vi "execute_trajectory_segment_final_point_only.vi"(6 "end time override":dbl=0.5, 8 "error in":errorcluster, 10 "in PathPlannerWayPoints":T1[](array[typedef]) {"HolonomicRotation"."SIN" format="%13.4f"; "HolonomicRotation"."COS" format="%13.4f"; "HolonomicRotation"."VALUE" format="%13.4f"; "NextControl"."Y" format="%14.3f"; "NextControl"."X" format="%14.3f"; "PrevControl"."Y" format="%14.3f"; "PrevControl"."X" format="%14.3f"; "AnchorPoint"."Y" format="%14.3f"; "AnchorPoint"."X" format="%14.3f"}, 11 "inHOLONOMIC_DRV_CTRL":T4={"poseTolerance"={"TRANSLATION"={"X"=0.0, "Y"=0.0}, "ROTATION"={"VALUE"=0.0, "COS"=1.0, "SIN"=0.0}}, "poseError"={"TRANSLATION"={"X"=0.0, "Y"=0.0}, "ROTATION"={"VALUE"=0.0, "COS"=1.0, "SIN"=0.0}}, "Enabled"=TRUE, "PID_xCtrl"={"Kp"=0.0, "Ki"=0.0, "Kd"=0.0, "Period"=0.0, "Max_Integral"=1.0, "Min_Integral"=-1.0, "Max_Input"=0.0, "Min_Input"=0.0, "Continuous"=FALSE, "PositionError"=0.0, "VelocityError"=0.0, "PrevError"=0.0, "TotalError"=0.0, "PositionTolerance"=0.05, "VelocityTolerance"=9.99e+35, "SetPoint"=0.0, "Kf"=0.0, "Prev_Deriv"=0.0, "Prev_Deriv 2"=0.0, "DerivativeFilter"=FALSE, "Min_Output"=-9.99e+35, "Max_Output"=9.9e+35, "Prev_F_P"=0.0, "Prev_F_P_2"=0.0, "AntiWindupActive"=FALSE, "Measurement"=0.0}, "PID_yCtrl"={"Kp"=0.0, "Ki"=0.0, "Kd"=0.0, "Period"=0.0, "Max_Integral"=1.0, "Min_Integral"=-1.0, "Max_Input"=0.0, "Min_Input"=0.0, "Continuous"=FALSE, "PositionError"=0.0, "VelocityError"=0.0, "PrevError"=0.0, "TotalError"=0.0, "PositionTolerance"=0.05, "VelocityTolerance"=9.99e+35, "SetPoint"=0.0, "Kf"=0.0, "Prev_Deriv"=0.0, "Prev_Deriv 2"=0.0, "DerivativeFilter"=FALSE, "Min_Output"=-9.99e+35, "Max_Output"=9.9e+35, "Prev_F_P"=0.0, "Prev_F_P_2"=0.0, "AntiWindupActive"=FALSE, "Measurement"=0.0}, "PROF_PID_thetaCtrl"={"Controller"={"Kp"=0.0, "Ki"=0.0, "Kd"=0.0, "Period"=0.0, "Max_Integral"=1.0, "Min_Integral"=-1.0, "Max_Input"=0.0, "Min_Input"=0.0, "Continuous"=FALSE, "PositionError"=0.0, "VelocityError"=0.0, "PrevError"=0.0, "TotalError"=0.0, "PositionTolerance"=0.05, "VelocityTolerance"=9.99e+35, "SetPoint"=0.0, "Kf"=0.0, "Prev_Deriv"=0.0, "Prev_Deriv 2"=0.0, "DerivativeFilter"=FALSE, "Min_Output"=-9.99e+35, "Max_Output"=9.9e+35, "Prev_F_P"=0.0, "Prev_F_P_2"=0.0, "AntiWindupActive"=FALSE, "Measurement"=0.0}, "Goal"={"Position"=0.0, "Velocity"=0.0}, "Setpoint"={"Position"=0.0, "Velocity"=0.0}, "Constraint"={"MaxVelocity"=0.0, "MaxAcceleration"=0.0}}, "RotationError"={"VALUE"=0.0, "COS"=1.0, "SIN"=0.0}, "FirstRun"=TRUE} {"RotationError"."SIN" format="%13.4f"; "RotationError"."COS" format="%13.4f"; "RotationError"."VALUE" format="%13.4f"; "PROF_PID_thetaCtrl"."Constraint"."MaxAcceleration" format="%16_6e"; "PROF_PID_thetaCtrl"."Constraint"."MaxVelocity" format="%16_6e"; "PROF_PID_thetaCtrl"."Setpoint"."Velocity" format="%16_6e"; "PROF_PID_thetaCtrl"."Setpoint"."Position" format="%16_6e"; "PROF_PID_thetaCtrl"."Goal"."Velocity" format="%16_6e"; "PROF_PID_thetaCtrl"."Goal"."Position" format="%16_6e"; "PROF_PID_thetaCtrl"."Controller"."Measurement" format="%16_6e"; "PROF_PID_thetaCtrl"."Controller"."Prev_F_P_2" format="%16_6e"; "PROF_PID_thetaCtrl"."Controller"."Prev_F_P" format="%16_6e"; "PROF_PID_thetaCtrl"."Controller"."Max_Output" format="%16_6e"; "PROF_PID_thetaCtrl"."Controller"."Min_Output" format="%16_6e"; "PROF_PID_thetaCtrl"."Controller"."Prev_Deriv 2" format="%16_6e"; "PROF_PID_thetaCtrl"."Controller"."Prev_Deriv" format="%16_6e"; "PROF_PID_thetaCtrl"."Controller"."Kf" format="%16_6e"; "PROF_PID_thetaCtrl"."Controller"."SetPoint" format="%16_6e"; "PROF_PID_thetaCtrl"."Controller"."VelocityTolerance" format="%16_6e"; "PROF_PID_thetaCtrl"."Controller"."PositionTolerance" format="%16_6e"; "PROF_PID_thetaCtrl"."Controller"."TotalError" format="%16_6e"; "PROF_PID_thetaCtrl"."Controller"."PrevError" format="%16_6e"; "PROF_PID_thetaCtrl"."Controller"."VelocityError" format="%16_6e"; "PROF_PID_thetaCtrl"."Controller"."PositionError" format="%16_6e"; "PROF_PID_thetaCtrl"."Controller"."Min_Input" format="%16_6e"; "PROF_PID_thetaCtrl"."Controller"."Max_Input" format="%16_6e"; "PROF_PID_thetaCtrl"."Controller"."Min_Integral" format="%16_6e"; "PROF_PID_thetaCtrl"."Controller"."Max_Integral" format="%16_6e"; "PROF_PID_thetaCtrl"."Controller"."Period" format="%16_6e"; "PROF_PID_thetaCtrl"."Controller"."Kd" format="%16_6e"; "PROF_PID_thetaCtrl"."Controller"."Ki" format="%16_6e"; "PROF_PID_thetaCtrl"."Controller"."Kp" format="%16_6e"; "PID_yCtrl"."Measurement" format="%16_6e"; "PID_yCtrl"."Prev_F_P_2" format="%16_6e"; "PID_yCtrl"."Prev_F_P" format="%16_6e"; "PID_yCtrl"."Max_Output" format="%16_6e"; "PID_yCtrl"."Min_Output" format="%16_6e"; "PID_yCtrl"."Prev_Deriv 2" format="%16_6e"; "PID_yCtrl"."Prev_Deriv" format="%16_6e"; "PID_yCtrl"."Kf" format="%16_6e"; "PID_yCtrl"."SetPoint" format="%16_6e"; "PID_yCtrl"."VelocityTolerance" format="%16_6e"; "PID_yCtrl"."PositionTolerance" format="%16_6e"; "PID_yCtrl"."TotalError" format="%16_6e"; "PID_yCtrl"."PrevError" format="%16_6e"; "PID_yCtrl"."VelocityError" format="%16_6e"; "PID_yCtrl"."PositionError" format="%16_6e"; "PID_yCtrl"."Min_Input" format="%16_6e"; "PID_yCtrl"."Max_Input" format="%16_6e"; "PID_yCtrl"."Min_Integral" format="%16_6e"; "PID_yCtrl"."Max_Integral" format="%16_6e"; "PID_yCtrl"."Period" format="%16_6e"; "PID_yCtrl"."Kd" format="%16_6e"; "PID_yCtrl"."Ki" format="%16_6e"; "PID_yCtrl"."Kp" format="%16_6e"; "PID_xCtrl"."Measurement" format="%16_6e"; "PID_xCtrl"."Prev_F_P_2" format="%16_6e"; "PID_xCtrl"."Prev_F_P" format="%16_6e"; "PID_xCtrl"."Max_Output" format="%16_6e"; "PID_xCtrl"."Min_Output" format="%16_6e"; "PID_xCtrl"."Prev_Deriv 2" format="%16_6e"; "PID_xCtrl"."Prev_Deriv" format="%16_6e"; "PID_xCtrl"."Kf" format="%16_6e"; "PID_xCtrl"."SetPoint" format="%16_6e"; "PID_xCtrl"."VelocityTolerance" format="%16_6e"; "PID_xCtrl"."PositionTolerance" format="%16_6e"; "PID_xCtrl"."TotalError" format="%16_6e"; "PID_xCtrl"."PrevError" format="%16_6e"; "PID_xCtrl"."VelocityError" format="%16_6e"; "PID_xCtrl"."PositionError" format="%16_6e"; "PID_xCtrl"."Min_Input" format="%16_6e"; "PID_xCtrl"."Max_Input" format="%16_6e"; "PID_xCtrl"."Min_Integral" format="%16_6e"; "PID_xCtrl"."Max_Integral" format="%16_6e"; "PID_xCtrl"."Period" format="%16_6e"; "PID_xCtrl"."Kd" format="%16_6e"; "PID_xCtrl"."Ki" format="%16_6e"; "PID_xCtrl"."Kp" format="%16_6e"; "poseError"."ROTATION"."SIN" format="%13.4f"; "poseError"."ROTATION"."COS" format="%13.4f"; "poseError"."ROTATION"."VALUE" format="%13.4f"; "poseError"."TRANSLATION"."Y" format="%14.3f"; "poseError"."TRANSLATION"."X" format="%14.3f"; "poseTolerance"."ROTATION"."SIN" format="%13.4f"; "poseTolerance"."ROTATION"."COS" format="%13.4f"; "poseTolerance"."ROTATION"."VALUE" format="%13.4f"; "poseTolerance"."TRANSLATION"."Y" format="%14.3f"; "poseTolerance"."TRANSLATION"."X" format="%14.3f"}) -> (0 "error out":errorcluster, 2 "out PathPlannerWayPoints":T1[](array[typedef]) {"HolonomicRotation"."SIN" format="%13.4f"; "HolonomicRotation"."COS" format="%13.4f"; "HolonomicRotation"."VALUE" format="%13.4f"; "NextControl"."Y" format="%14.3f"; "NextControl"."X" format="%14.3f"; "PrevControl"."Y" format="%14.3f"; "PrevControl"."X" format="%14.3f"; "AnchorPoint"."Y" format="%14.3f"; "AnchorPoint"."X" format="%14.3f"}, 3 "outHOLONOMIC_DRV_CTRL":T4={"poseTolerance"={"TRANSLATION"={"X"=0.0, "Y"=0.0}, "ROTATION"={"VALUE"=0.0, "COS"=1.0, "SIN"=0.0}}, "poseError"={"TRANSLATION"={"X"=0.0, "Y"=0.0}, "ROTATION"={"VALUE"=0.0, "COS"=1.0, "SIN"=0.0}}, "Enabled"=TRUE, "PID_xCtrl"={"Kp"=0.0, "Ki"=0.0, "Kd"=0.0, "Period"=0.0, "Max_Integral"=1.0, "Min_Integral"=-1.0, "Max_Input"=0.0, "Min_Input"=0.0, "Continuous"=FALSE, "PositionError"=0.0, "VelocityError"=0.0, "PrevError"=0.0, "TotalError"=0.0, "PositionTolerance"=0.05, "VelocityTolerance"=9.99e+35, "SetPoint"=0.0, "Kf"=0.0, "Prev_Deriv"=0.0, "Prev_Deriv 2"=0.0, "DerivativeFilter"=FALSE, "Min_Output"=-9.99e+35, "Max_Output"=9.9e+35, "Prev_F_P"=0.0, "Prev_F_P_2"=0.0, "AntiWindupActive"=FALSE, "Measurement"=0.0}, "PID_yCtrl"={"Kp"=0.0, "Ki"=0.0, "Kd"=0.0, "Period"=0.0, "Max_Integral"=1.0, "Min_Integral"=-1.0, "Max_Input"=0.0, "Min_Input"=0.0, "Continuous"=FALSE, "PositionError"=0.0, "VelocityError"=0.0, "PrevError"=0.0, "TotalError"=0.0, "PositionTolerance"=0.05, "VelocityTolerance"=9.99e+35, "SetPoint"=0.0, "Kf"=0.0, "Prev_Deriv"=0.0, "Prev_Deriv 2"=0.0, "DerivativeFilter"=FALSE, "Min_Output"=-9.99e+35, "Max_Output"=9.9e+35, "Prev_F_P"=0.0, "Prev_F_P_2"=0.0, "AntiWindupActive"=FALSE, "Measurement"=0.0}, "PROF_PID_thetaCtrl"={"Controller"={"Kp"=0.0, "Ki"=0.0, "Kd"=0.0, "Period"=0.0, "Max_Integral"=1.0, "Min_Integral"=-1.0, "Max_Input"=0.0, "Min_Input"=0.0, "Continuous"=FALSE, "PositionError"=0.0, "VelocityError"=0.0, "PrevError"=0.0, "TotalError"=0.0, "PositionTolerance"=0.05, "VelocityTolerance"=9.99e+35, "SetPoint"=0.0, "Kf"=0.0, "Prev_Deriv"=0.0, "Prev_Deriv 2"=0.0, "DerivativeFilter"=FALSE, "Min_Output"=-9.99e+35, "Max_Output"=9.9e+35, "Prev_F_P"=0.0, "Prev_F_P_2"=0.0, "AntiWindupActive"=FALSE, "Measurement"=0.0}, "Goal"={"Position"=0.0, "Velocity"=0.0}, "Setpoint"={"Position"=0.0, "Velocity"=0.0}, "Constraint"={"MaxVelocity"=0.0, "MaxAcceleration"=0.0}}, "RotationError"={"VALUE"=0.0, "COS"=1.0, "SIN"=0.0}, "FirstRun"=TRUE} {"RotationError"."SIN" format="%13.4f"; "RotationError"."COS" format="%13.4f"; "RotationError"."VALUE" format="%13.4f"; "PROF_PID_thetaCtrl"."Constraint"."MaxAcceleration" format="%16_6e"; "PROF_PID_thetaCtrl"."Constraint"."MaxVelocity" format="%16_6e"; "PROF_PID_thetaCtrl"."Setpoint"."Velocity" format="%16_6e"; "PROF_PID_thetaCtrl"."Setpoint"."Position" format="%16_6e"; "PROF_PID_thetaCtrl"."Goal"."Velocity" format="%16_6e"; "PROF_PID_thetaCtrl"."Goal"."Position" format="%16_6e"; "PROF_PID_thetaCtrl"."Controller"."Measurement" format="%16_6e"; "PROF_PID_thetaCtrl"."Controller"."Prev_F_P_2" format="%16_6e"; "PROF_PID_thetaCtrl"."Controller"."Prev_F_P" format="%16_6e"; "PROF_PID_thetaCtrl"."Controller"."Max_Output" format="%16_6e"; "PROF_PID_thetaCtrl"."Controller"."Min_Output" format="%16_6e"; "PROF_PID_thetaCtrl"."Controller"."Prev_Deriv 2" format="%16_6e"; "PROF_PID_thetaCtrl"."Controller"."Prev_Deriv" format="%16_6e"; "PROF_PID_thetaCtrl"."Controller"."Kf" format="%16_6e"; "PROF_PID_thetaCtrl"."Controller"."SetPoint" format="%16_6e"; "PROF_PID_thetaCtrl"."Controller"."VelocityTolerance" format="%16_6e"; "PROF_PID_thetaCtrl"."Controller"."PositionTolerance" format="%16_6e"; "PROF_PID_thetaCtrl"."Controller"."TotalError" format="%16_6e"; "PROF_PID_thetaCtrl"."Controller"."PrevError" format="%16_6e"; "PROF_PID_thetaCtrl"."Controller"."VelocityError" format="%16_6e"; "PROF_PID_thetaCtrl"."Controller"."PositionError" format="%16_6e"; "PROF_PID_thetaCtrl"."Controller"."Min_Input" format="%16_6e"; "PROF_PID_thetaCtrl"."Controller"."Max_Input" format="%16_6e"; "PROF_PID_thetaCtrl"."Controller"."Min_Integral" format="%16_6e"; "PROF_PID_thetaCtrl"."Controller"."Max_Integral" format="%16_6e"; "PROF_PID_thetaCtrl"."Controller"."Period" format="%16_6e"; "PROF_PID_thetaCtrl"."Controller"."Kd" format="%16_6e"; "PROF_PID_thetaCtrl"."Controller"."Ki" format="%16_6e"; "PROF_PID_thetaCtrl"."Controller"."Kp" format="%16_6e"; "PID_yCtrl"."Measurement" format="%16_6e"; "PID_yCtrl"."Prev_F_P_2" format="%16_6e"; "PID_yCtrl"."Prev_F_P" format="%16_6e"; "PID_yCtrl"."Max_Output" format="%16_6e"; "PID_yCtrl"."Min_Output" format="%16_6e"; "PID_yCtrl"."Prev_Deriv 2" format="%16_6e"; "PID_yCtrl"."Prev_Deriv" format="%16_6e"; "PID_yCtrl"."Kf" format="%16_6e"; "PID_yCtrl"."SetPoint" format="%16_6e"; "PID_yCtrl"."VelocityTolerance" format="%16_6e"; "PID_yCtrl"."PositionTolerance" format="%16_6e"; "PID_yCtrl"."TotalError" format="%16_6e"; "PID_yCtrl"."PrevError" format="%16_6e"; "PID_yCtrl"."VelocityError" format="%16_6e"; "PID_yCtrl"."PositionError" format="%16_6e"; "PID_yCtrl"."Min_Input" format="%16_6e"; "PID_yCtrl"."Max_Input" format="%16_6e"; "PID_yCtrl"."Min_Integral" format="%16_6e"; "PID_yCtrl"."Max_Integral" format="%16_6e"; "PID_yCtrl"."Period" format="%16_6e"; "PID_yCtrl"."Kd" format="%16_6e"; "PID_yCtrl"."Ki" format="%16_6e"; "PID_yCtrl"."Kp" format="%16_6e"; "PID_xCtrl"."Measurement" format="%16_6e"; "PID_xCtrl"."Prev_F_P_2" format="%16_6e"; "PID_xCtrl"."Prev_F_P" format="%16_6e"; "PID_xCtrl"."Max_Output" format="%16_6e"; "PID_xCtrl"."Min_Output" format="%16_6e"; "PID_xCtrl"."Prev_Deriv 2" format="%16_6e"; "PID_xCtrl"."Prev_Deriv" format="%16_6e"; "PID_xCtrl"."Kf" format="%16_6e"; "PID_xCtrl"."SetPoint" format="%16_6e"; "PID_xCtrl"."VelocityTolerance" format="%16_6e"; "PID_xCtrl"."PositionTolerance" format="%16_6e"; "PID_xCtrl"."TotalError" format="%16_6e"; "PID_xCtrl"."PrevError" format="%16_6e"; "PID_xCtrl"."VelocityError" format="%16_6e"; "PID_xCtrl"."PositionError" format="%16_6e"; "PID_xCtrl"."Min_Input" format="%16_6e"; "PID_xCtrl"."Max_Input" format="%16_6e"; "PID_xCtrl"."Min_Integral" format="%16_6e"; "PID_xCtrl"."Max_Integral" format="%16_6e"; "PID_xCtrl"."Period" format="%16_6e"; "PID_xCtrl"."Kd" format="%16_6e"; "PID_xCtrl"."Ki" format="%16_6e"; "PID_xCtrl"."Kp" format="%16_6e"; "poseError"."ROTATION"."SIN" format="%13.4f"; "poseError"."ROTATION"."COS" format="%13.4f"; "poseError"."ROTATION"."VALUE" format="%13.4f"; "poseError"."TRANSLATION"."Y" format="%14.3f"; "poseError"."TRANSLATION"."X" format="%14.3f"; "poseTolerance"."ROTATION"."SIN" format="%13.4f"; "poseTolerance"."ROTATION"."COS" format="%13.4f"; "poseTolerance"."ROTATION"."VALUE" format="%13.4f"; "poseTolerance"."TRANSLATION"."Y" format="%14.3f"; "poseTolerance"."TRANSLATION"."X" format="%14.3f"})   [LabVIEW 2020]
doc: "Executes the next segment of a <B>PathPlanner</B> trajectory."
uses:
  <vilib>/Rock Robotics/WPI/ThirdParty/MJansen/PathPlanner/PathPlannerWaypoint.ctl
  <vilib>/Rock Robotics/WPI/ThirdParty/JAS_Junk/TrajLib/TRANSLATION2D.ctl
  <vilib>/Rock Robotics/WPI/ThirdParty/JAS_Junk/TrajLib/ROTATION2D.ctl
  <vilib>/Rock Robotics/WPI/ThirdParty/JAS_Junk/TrajLib/HOLONOMIC_DRV_CTRL.ctl
  <vilib>/Rock Robotics/WPI/ThirdParty/JAS_Junk/TrajLib/POSE2D.ctl
  <vilib>/Rock Robotics/WPI/ThirdParty/JAS_Junk/TrajLib/PID_CONTROLLER.ctl
  <vilib>/Rock Robotics/WPI/ThirdParty/JAS_Junk/TrajLib/PROFILED_PID_CONTROLLER.ctl
  <vilib>/Rock Robotics/WPI/ThirdParty/JAS_Junk/TrajLib/TRAPEZOID_PROFILE_STATE.ctl
  <vilib>/Rock Robotics/WPI/ThirdParty/JAS_Junk/TrajLib/TRAPEZOID_PROFILE_CONSTRAINT.ctl
  <vilib>/Rock Robotics/WPI/ThirdParty/JAS_Junk/TrajLib/HolDrvCtrl_Calculate.vi
  <vilib>/Rock Robotics/WPI/ThirdParty/JAS_Junk/TrajLib/ProfiledPIDController_Calculate_Meas_Goal.vi
  <vilib>/Rock Robotics/WPI/ThirdParty/JAS_Junk/TrajLib/ChassisSpeeds_FromFieldRelativeSpeeds.vi
  <vilib>/Rock Robotics/WPI/ThirdParty/JAS_Junk/TrajLib/PIDController_Reset.vi
  <vilib>/Rock Robotics/WPI/ThirdParty/JAS_Junk/TrajLib/PIDController_Calculate_SP_PV.vi
  <vilib>/Rock Robotics/WPI/ThirdParty/JAS_Junk/TrajLib/ProfiledPIDController_Reset_PosOnly.vi
  <vilib>/Rock Robotics/WPI/ThirdParty/JAS_Junk/TrajLib/Pose_getXYAngle.vi
  <vilib>/Rock Robotics/WPI/ThirdParty/JAS_Junk/TrajLib/Rotation_GetAngleCosSin.vi
  <vilib>/Rock Robotics/WPI/ThirdParty/JAS_Junk/TrajLib/Pose_RelativeTo.vi
  <vilib>/Rock Robotics/WPI/ThirdParty/JAS_Junk/TrajLib/Pose_getRotation.vi
  <vilib>/Rock Robotics/WPI/ThirdParty/JAS_Junk/TrajLib/Rotation_Minus.vi
  <vilib>/Rock Robotics/WPI/ThirdParty/JAS_Junk/TrajLib/ProfiledPIDController_SetGoal_PosOnly.vi
  <vilib>/Rock Robotics/WPI/ThirdParty/JAS_Junk/TrajLib/ProfiledPIDController_Calculate_Meas.vi
  <vilib>/Rock Robotics/WPI/ThirdParty/JAS_Junk/TrajLib/Rotation_GetCos.vi
  <vilib>/Rock Robotics/WPI/ThirdParty/JAS_Junk/TrajLib/Rotation_GetSin.vi
  <vilib>/Rock Robotics/WPI/ThirdParty/JAS_Junk/TrajLib/ChassisSpeeds_New.vi
  <vilib>/Rock Robotics/WPI/ThirdParty/JAS_Junk/TrajLib/PIDController_SetSetpoint.vi
  <vilib>/Rock Robotics/WPI/ThirdParty/JAS_Junk/TrajLib/PIDController_Calculate_PV.vi
  <vilib>/Rock Robotics/WPI/ThirdParty/JAS_Junk/TrajLib/TrapProfState_New.vi
  <vilib>/Rock Robotics/WPI/ThirdParty/JAS_Junk/TrajLib/ProfiledPIDController_Reset.vi
  <vilib>/Rock Robotics/WPI/ThirdParty/JAS_Junk/TrajLib/Transform_Create_PosePose.vi
  <vilib>/Rock Robotics/WPI/ThirdParty/JAS_Junk/TrajLib/Pose_New_TRRO.vi
  <vilib>/Rock Robotics/WPI/ThirdParty/JAS_Junk/TrajLib/Rotation_UnaryMinus.vi
  <vilib>/Rock Robotics/WPI/ThirdParty/JAS_Junk/TrajLib/Rotation_RotateBy.vi
  <vilib>/Rock Robotics/WPI/ThirdParty/JAS_Junk/TrajLib/ProfiledPIDController_SetGoal.vi
  <vilib>/Rock Robotics/WPI/ThirdParty/JAS_Junk/TrajLib/TrapProfile_New.vi
  <vilib>/Rock Robotics/WPI/ThirdParty/JAS_Junk/TrajLib/ProfiledPIDController_GetPeriod.vi
  <vilib>/Rock Robotics/WPI/ThirdParty/JAS_Junk/TrajLib/TrapProfile_Calculate.vi
  <vilib>/Rock Robotics/WPI/ThirdParty/JAS_Junk/TrajLib/ControllerUtil_GetModulusError.vi
  <vilib>/Rock Robotics/WPI/ThirdParty/JAS_Junk/TrajLib/Translation_RotateBy.vi
  <vilib>/Rock Robotics/WPI/ThirdParty/JAS_Junk/TrajLib/Translation_Minus.vi
  <vilib>/Rock Robotics/WPI/ThirdParty/JAS_Junk/TrajLib/Rotation_CreateAngle.vi
  <vilib>/Rock Robotics/WPI/ThirdParty/JAS_Junk/TrajLib/Rotation_CreateXY.vi
  <vilib>/Rock Robotics/WPI/ThirdParty/JAS_Junk/TrajLib/TrapProfile_ShouldFlipAcceleration.vi
  <vilib>/Rock Robotics/WPI/ThirdParty/JAS_Junk/TrajLib/TrapProfile_Direct.vi
  <vilib>/Rock Robotics/SystemInterfaces/NetworkCommunication/NetComm_UsageReport_report.vi
  <vilib>/Rock Robotics/WPI/ThirdParty/JAS_Junk/TrajLib/PIDController_GetPeriod.vi
  <vilib>/Rock Robotics/WPI/ThirdParty/JAS_Junk/TrajLib/Translation_Create.vi
  <vilib>/Rock Robotics/WPI/ThirdParty/JAS_Junk/TrajLib/Util_CalcDist.vi
  <vilib>/Utility/semaphor.llb/Obtain Semaphore Reference.vi
  <vilib>/Rock Robotics/WPI/ThirdParty/JAS_Junk/TrajLib/Timer_Reset.vi
  Robot Global Data.vi
  <vilib>/Utility/error.llb/Error Cluster From Error Code.vi
  Subsystems/Swerve/swerve_globals.vi
  <vilib>/Rock Robotics/WPI/ThirdParty/JAS_Junk/TrajLib/Util_LibraryGlobals.vi
  <vilib>/ErrorRing/Error Ring.xnode
  <vilib>/Rock Robotics/WPI/ThirdParty/JAS_Junk/TrajLib/Trajectory_Library.lvlib
  <vilib>/Rock Robotics/WPI/ThirdParty/MJansen/PathPlanner/PathPlanner.lvlib
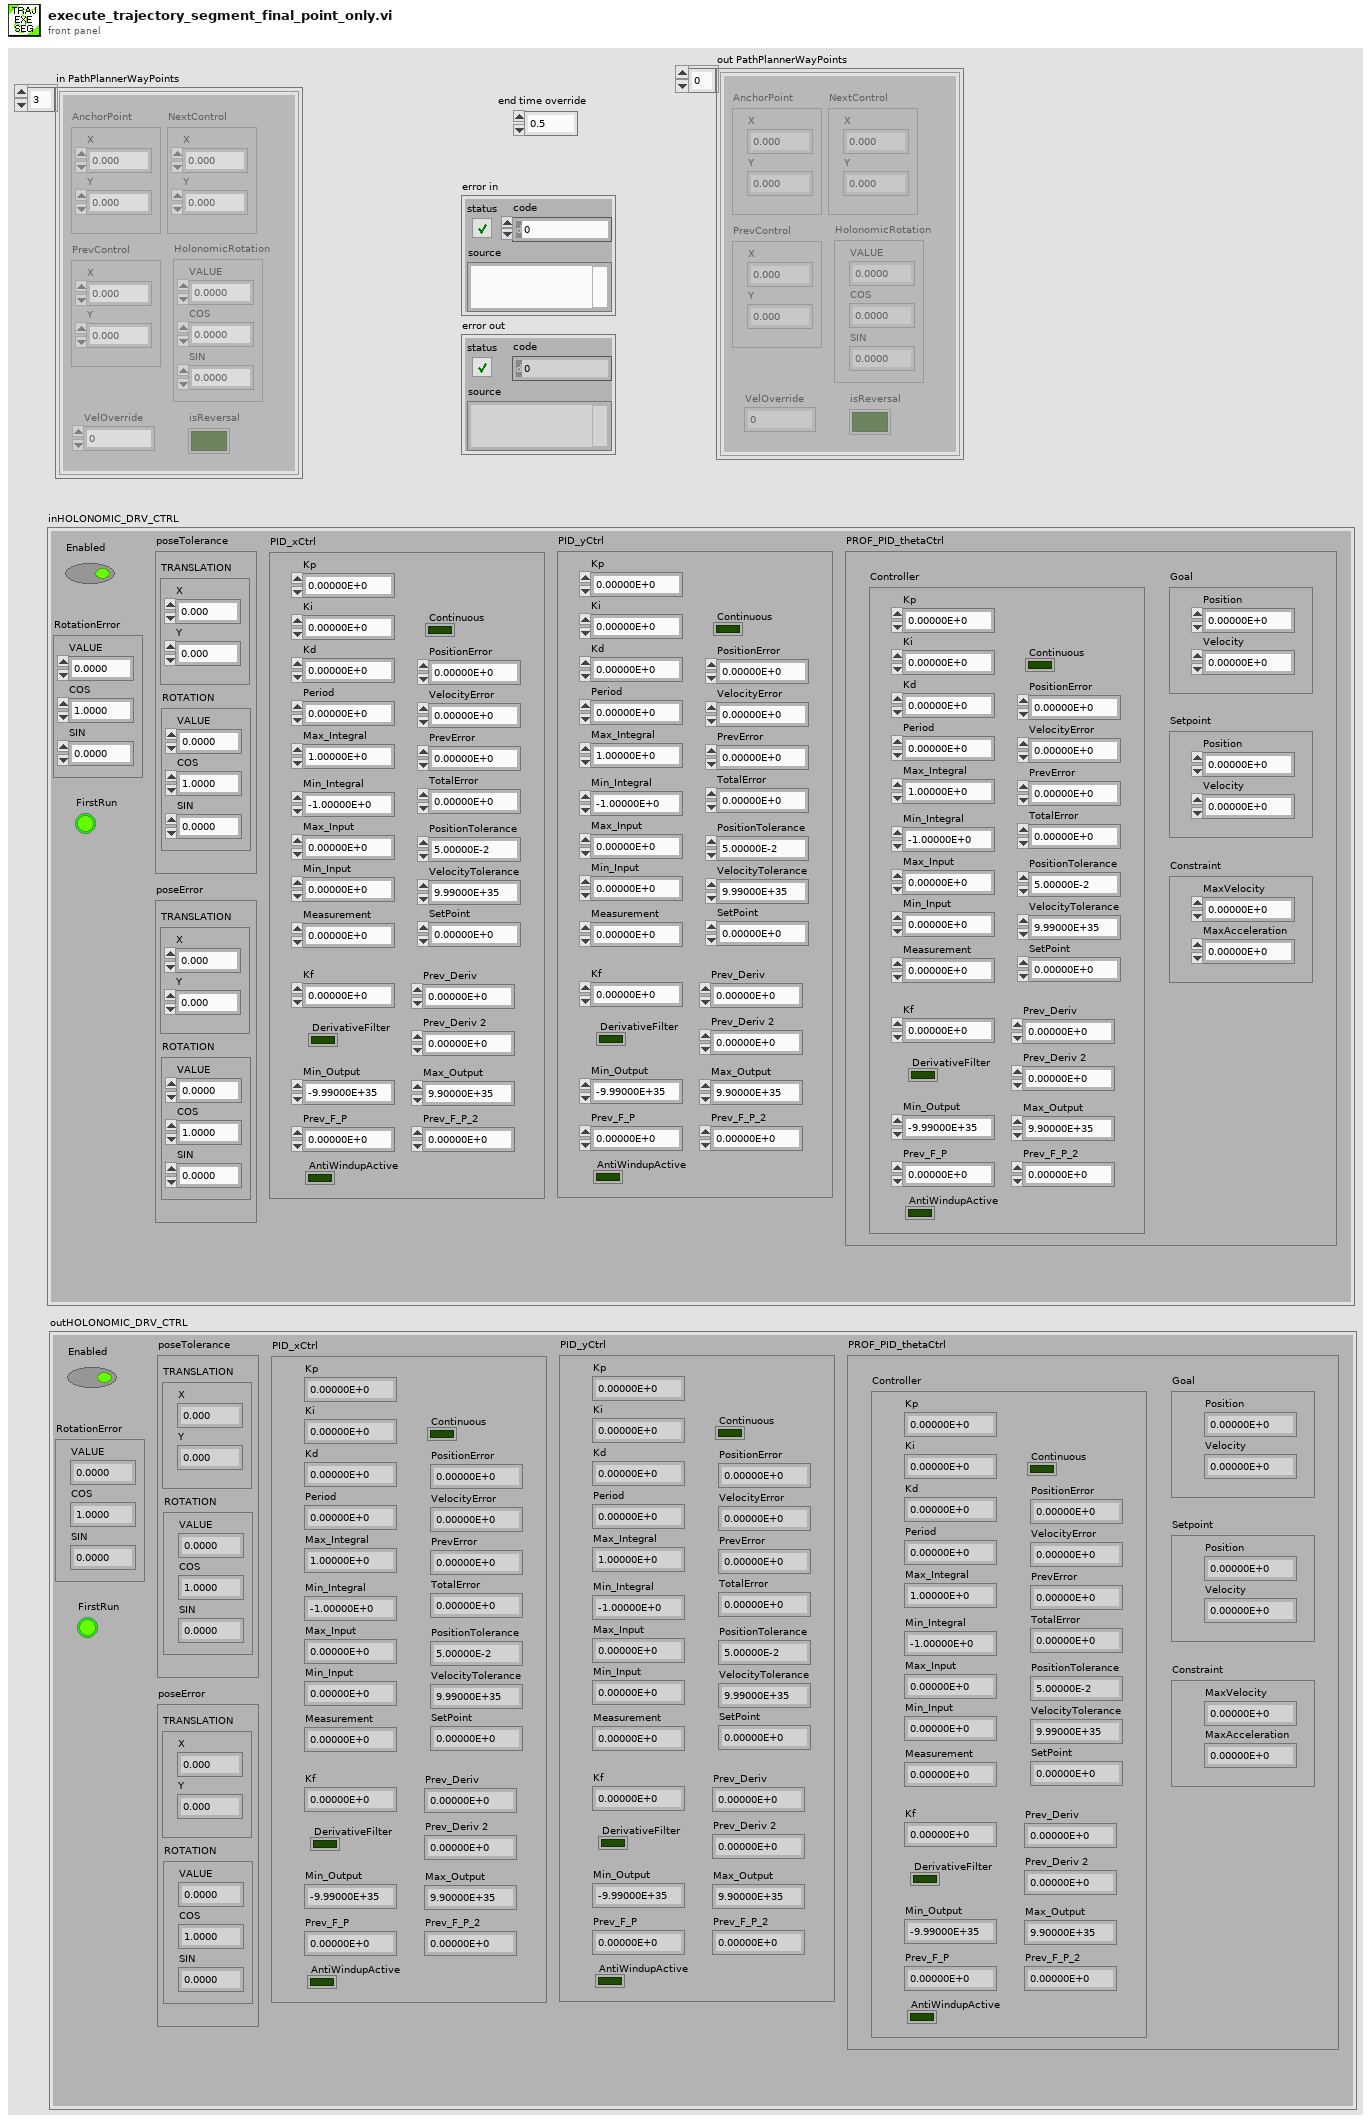
[diagram p1: front panel]
types:
  T1 = typedef "PathPlanner.lvlib/PathPlannerWaypoint.ctl" = cluster{"AnchorPoint":T2, "PrevControl":T2, "NextControl":T2, "HolonomicRotation":T3, "VelOverride":dbl, "isReversal":bool}
  T2 = typedef "Trajectory_Library.lvlib/TRANSLATION2D.ctl" = cluster{"X":dbl, "Y":dbl}
  T3 = typedef "Trajectory_Library.lvlib/ROTATION2D.ctl" = cluster{"VALUE":dbl, "COS":dbl, "SIN":dbl}
  T4 = typedef "Trajectory_Library.lvlib/HOLONOMIC_DRV_CTRL.ctl" = cluster{"poseTolerance":T5, "poseError":T5, "Enabled":bool, "PID_xCtrl":T6, "PID_yCtrl":T6, "PROF_PID_thetaCtrl":T7, "RotationError":T3, "FirstRun":bool}
  T5 = typedef "Trajectory_Library.lvlib/POSE2D.ctl" = cluster{"TRANSLATION":T2, "ROTATION":T3}
  T6 = typedef "Trajectory_Library.lvlib/PID_CONTROLLER.ctl" = cluster{"Kp":dbl, "Ki":dbl, "Kd":dbl, "Period":dbl, "Max_Integral":dbl, "Min_Integral":dbl, "Max_Input":dbl, "Min_Input":dbl, "Continuous":bool, "PositionError":dbl, "VelocityError":dbl, "PrevError":dbl, "TotalError":dbl, "PositionTolerance":dbl, "VelocityTolerance":dbl, "SetPoint":dbl, "Kf":dbl, "Prev_Deriv":dbl, "Prev_Deriv 2":dbl, "DerivativeFilter":bool, "Min_Output":dbl, "Max_Output":dbl, "Prev_F_P":dbl, "Prev_F_P_2":dbl, "AntiWindupActive":bool, "Measurement":dbl}
  T7 = typedef "Trajectory_Library.lvlib/PROFILED_PID_CONTROLLER.ctl" = cluster{"Controller":T6, "Goal":T8, "Setpoint":T8, "Constraint":T9}
  T8 = typedef "Trajectory_Library.lvlib/TRAPEZOID_PROFILE_STATE.ctl" = cluster{"Position":dbl, "Velocity":dbl}
  T9 = typedef "Trajectory_Library.lvlib/TRAPEZOID_PROFILE_CONSTRAINT.ctl" = cluster{"MaxVelocity":dbl, "MaxAcceleration":dbl}
  T10 = typedef "Trajectory_Library.lvlib/TIMER.ctl" = cluster{"StartTime":dbl, "Accumulated TIme":dbl, "Running":bool, "semaphore":T11}
  T11 = typedef "Semaphore RefNum" = refnum<k1>
  T12 = typedef "PathPlanner.lvlib/PathPlannerTrajectory.ctl" = cluster{"TotalTimeSeconds":dbl, "States":T13[]}
  T13 = typedef "PathPlanner.lvlib/PathPlannerState.ctl" = cluster{"AngularAcceleration":T3, "PositionMeters":dbl, "TrajectoryState":T14, "AngularVelocity":T3, "HolonomicRotation":T3, "CurveRadius":dbl, "DeltaPos":dbl}
  T14 = typedef "Trajectory_Library.lvlib/TRAJ_STATE.ctl" = cluster{"TimeSeconds":dbl, "Velocity":dbl, "Acceleration":dbl, "POSE":T5, "Curvature":dbl}
  T15 = typedef "Trajectory_Library.lvlib/CHASSIS_SPEEDS.ctl" = cluster{"vX":dbl, "vY":dbl, "vOmega":dbl}
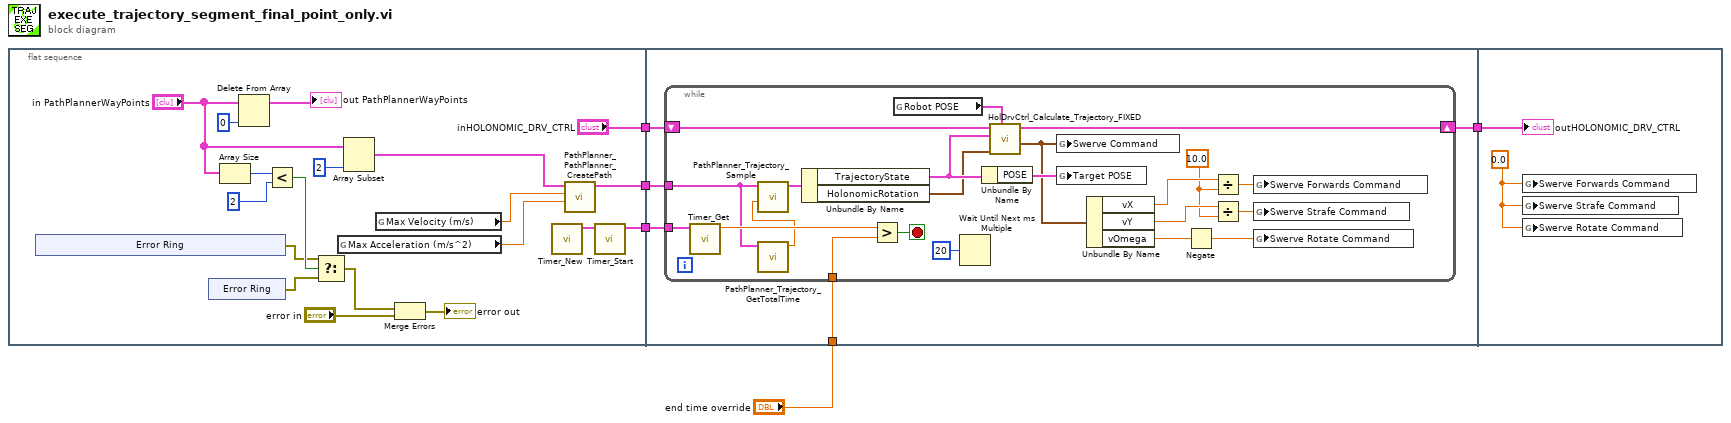
[diagram p0: block diagram]
diagram:
  n1 = flat-sequence {
    tunnel: [w6] -> w4
    tunnel: [w7] -> w3
    tunnel: ["inHOLONOMIC_DRV_CTRL"] -> w2
    tunnel: [w31] -> w5
    tunnel: w4 -> [w34]
    tunnel: w3 -> [w33]
    tunnel: w2 -> [w32]
    tunnel: "end time override" -> [w30]
    tunnel: w5 -> [w57]
    frame #0 {
      n2 = xnode "Error Ring"() -> ("error out"=w16:errorcluster)
      n3 = xnode "Error Ring"() -> ("error out"=w17:errorcluster)
      n4 = Array Size(array="in PathPlannerWayPoints") -> (size(s)=w21:i32)
      n5 = Delete From Array(array="in PathPlannerWayPoints", index=0) -> (array with subset deleted=→"out PathPlannerWayPoints":T1[])  [unwired: 1 in, 1 out]
      n6 = Less?(x=w21, y=2) -> (x < y?=w24:bool)
      n7 = Select(t=w16, s=w24, f=w17) -> (s? t:f=w19:errorcluster)
      n8 = global read "Robot Global Data.vi" "Max Acceleration (m/s^2)"() -> (w15:dbl)
      n9 = Array Subset(array="in PathPlannerWayPoints", length=2) -> (w12:T1[])  [unwired: 1 in]
      n10 = global read "Robot Global Data.vi" "Max Velocity (m/s)"() -> (w14:dbl)
      n11 = Merge Errors(w19, "error in") -> (→"error out":errorcluster)
      n12 = call <vilib>:"Timer_New.vi"() -> ("TIMER"=w13:T10)  [unwired: 11 in]
      n13 = call <vilib>:"PathPlanner_PathPlanner_CreatePath.vi"("MaxAcceleration"=w15, "MaxVelocity"=w14, "PathPlannerWayPoints"=w12) -> ("PathPlannerTrajectory"=w7:T12)  [unwired: 8 in]
      n14 = call <vilib>:"Timer_Start.vi"("in Timer"=w13) -> ("out Timer"=w6:T10)  [unwired: 10 in]
    }
    frame #1 {
      n15 = while {
        tunnel: w34 -> [w56]
        shift-right: [w43] -> w31
        shift-left: w32 -> [w53]
        tunnel: w33 -> [w42]
        tunnel: w30 -> [w36]
        stop <- w41 stop-if-true
        w44 = 10.0 ("y")
        n16 = call <vilib>:"Timer_Get.vi"("TIMER"=w56) -> ("CurrentTImer"=w51:dbl)  [unwired: 10 in]
        n17 = call <vilib>:"PathPlanner_Trajectory_GetTotalTime.vi"("PathPlannerTrajectory"=w42) -> ("TotalTimeSeconds"=w35:dbl)  [unwired: 10 in]
        n18 = call <vilib>:"PathPlanner_Trajectory_Sample.vi"("Time"=w35, "PathPlannerTrajectory"=w42) -> ("PathPlannerState"=w55:T13)  [unwired: 9 in]
        n19 = Unbundle By Name(w55) -> ("TrajectoryState"=w40:T14, "HolonomicRotation"=w39:T3)
        n20 = Greater?(x=w51, y=w36) -> (0:w41:bool)
        n21 = global read "swerve_globals.vi" "Robot POSE"() -> (w54:T5)
        n22 = Wait Until Next ms Multiple(millisecond multiple=u32 20) -> ()  [unwired: 1 out]
        n23 = Unbundle By Name(w40) -> ("POSE"=w50:T5)
        n24 = call "HolDrvCtrl_Calculate_Trajectory_FIXED.vi"("currentPose"=w54, "angleRef"=w39, "desiredTrajState"=w40, "inHOLONOMIC_DRV_CTRL"=w53) -> ("calcChassisSpeed"=w49:T15, "outHOLONOMIC_DRV_CTRL"=w43:T4)  [unwired: 6 in]
        n25 = global write "swerve_globals.vi" "Swerve Command"(w49) -> ()
        n26 = global write "swerve_globals.vi" "Target POSE"(w50) -> ()
        n27 = Unbundle By Name(w49) -> ("vX"=w48:dbl, "vY"=w47:dbl, "vOmega"=w38:dbl)
        n28 = Negate(x=w38) -> (-x=w37:dbl)
        n29 = Divide(x=w48, y=w44) -> (x/y=w45:dbl)
        n30 = Divide(x=w47, y=w44) -> (x/y=w46:dbl)
        n31 = global write "swerve_globals.vi" "Swerve Forwards Command"(w45) -> ()
        n32 = global write "swerve_globals.vi" "Swerve Strafe Command"(w46) -> ()
        n33 = global write "swerve_globals.vi" "Swerve Rotate Command"(w37) -> ()
      }
    }
    frame #2 {
      w58 = 0.0 ("Swerve Forwards Command")
      n34 = global write "swerve_globals.vi" "Swerve Forwards Command"(w58) -> ()
      n35 = global write "swerve_globals.vi" "Swerve Strafe Command"(w58) -> ()
      n36 = global write "swerve_globals.vi" "Swerve Rotate Command"(w58) -> ()
      "outHOLONOMIC_DRV_CTRL" <- w57
    }
  }
